vi "HexToDword.vi"(11 "数组":u16[](array[numeric]) format="%04xH") -> (3 "DWORD":i32[](array[numeric]))   [LabVIEW 2016, in "PLC.lvlib"]
uses:
  PLC.lvlib
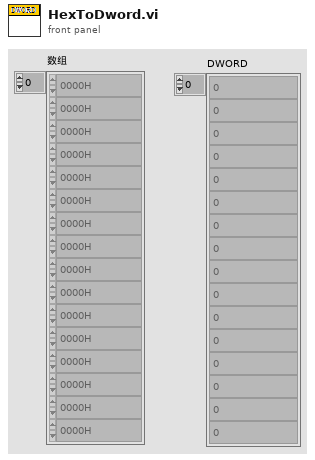
[diagram p1: front panel]
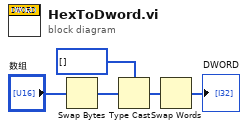
[diagram p0: block diagram]
diagram:
  n1 = Swap Bytes(anything="数组") -> (byte swapped=w4:u16[])
  n2 = Type Cast(type=i32[] [], x=w4) -> (*(type *) &x=w2:i32[])
  n3 = Swap Words(1:w2) -> (0:→"DWORD":i32[])
